vi "UtilityLib.align string.vi"(2 "stringIn":string, 3 "stringLength (80)":i32=80, 5 "error in (no error)":errorcluster) -> (16 "stringOut":string, 19 "error out":errorcluster)   [LabVIEW 2014, in "UtilityLib.lvlib"]
doc: "Aligns a string to the specified length by truncating it or by filling it up with \"\\0\".\n\nLicense Agreement for this software:\n\nCopyright (C)\nGesellschaft für Schwerionenforschung, GSI\nPlanckstr. 1\n64291 Darmstadt\nGermany\n\nContact: D.Beck@gsi.de \n\nThis program is free software; you can redistribute it and/or modify it under the terms of the GNU General Public License as published by the Free Software Foundation; either version 2 of the license, or (at your option) any later version.\n\nThis program is distributed in the hope that it will be useful, but WITHOUT ANY WARRANTY; without even the implied warranty of MERCHANTABILITY or FITNESS FOR A PARTICULAR PURPOSE. See the GNU General License for more details (http://www.gnu.org).\n\nGesellschaft für Schwerionenforschung, GSI\nPlanckstr. 1, 64291 Darmstadt, Germany\nFor all questions and ideas contact: M.Richter@gsi.de, H.Brand@gsi.de or D.Beck@gsi.de.\nLast update: 17-JUN-2004"
uses:
  UtilityLib.lvlib
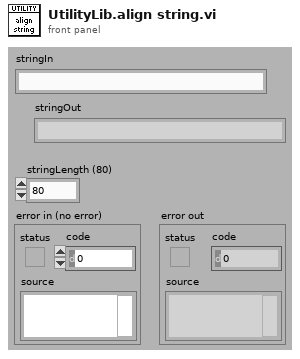
[diagram p1: front panel]
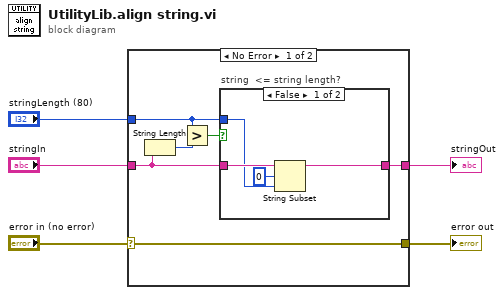
[diagram p0: block diagram]
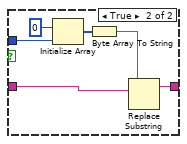
[diagram p2: hidden frame]
diagram:
  n1 = case shown="No Error" "error in (no error)" {
    selector: "error in (no error)" -> [w11 w23]
    tunnel: [w11 w23] -> w4
    tunnel: "stringIn" -> [w8 w22]
    tunnel: "stringLength (80)" -> [w7 _]
    tunnel: [w6 w22] -> w1
    frame No Error {
      n2 = String Length(string=w8) -> (length=w10:i32)
      n3 = Greater?(x=w7, y=w10) -> (0:w9:bool)
      n4 = case "string  <= string length?" shown="False" w9 {
        tunnel: w8 -> [w15 w16]
        tunnel: w7 -> [w13 w21]
        tunnel: [w12 w18] -> w6
        frame False {
          n5 = String Subset(string=w15, offset (0)=0, length (rest)=w13) -> (substring=w12:string)
        }
        frame True {
          n6 = Initialize Array(u8 0, w21) -> (w19:u8[])
          n7 = Byte Array To String(unsigned byte array=w19) -> (string=w17:string)
          n8 = Replace Substring(4:w16, 5:w17) -> (1:w18:string)  [unwired: 2 in, 1 out]
        }
      }
    }
    frame Error {
    }
  }
  "error out" <- w4
  "stringOut" <- w1
